vi "sub1.vi"() -> ()   [LabVIEW 2018]
uses:
  global_variable.vi
panel:
  in  "숫자형 컨트롤":dbl
  in  "정지버튼":bool
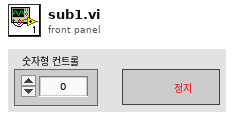
[diagram p1: front panel]
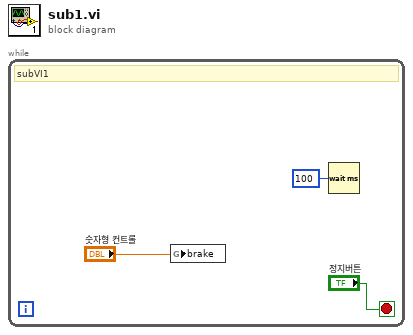
[diagram p0: block diagram]
diagram:
  n1 = while {
    stop <- "정지버튼" stop-if-true
    # "subVI1"
    n2 = global write "global_variable.vi" "brake"("숫자형 컨트롤") -> ()
    n3 = Wait (ms)(milliseconds to wait=u32 100 ("대기 시간 (ms)")) -> ()  [unwired: 1 out]
  }
